vi "update_json_by_inserting_array.vi"(9 "json_to_insert_to_array(from recursive output)":string, 10 "ori_json_array":string[](array[string]), 11 "original_json":string) -> (3 "<JSON>输出":string)   [LabVIEW 2020]
uses:
  <vilib>/JDP Science/JSONtext/support/Format JSON Array Text.vi
  <vilib>/JDP Science/JSONtext/JSONtext.lvlib
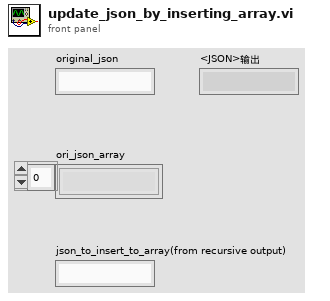
[diagram p1: front panel]
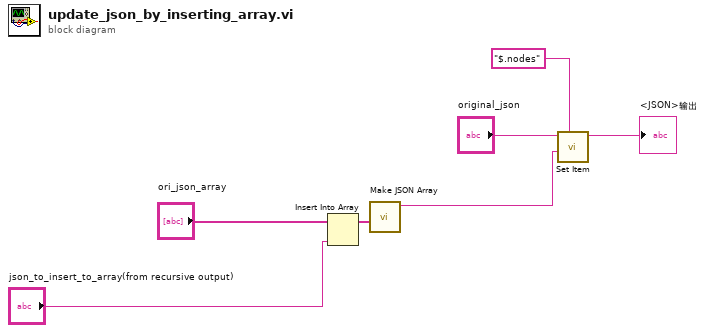
[diagram p0: block diagram]
diagram:
  n1 = Insert Into Array(array="ori_json_array", new element="json_to_insert_to_array(from recursive output)") -> (w2:string[])  [unwired: 1 in]
  n2 = call <vilib>:"Make JSON Array.vi"("JSON Elements"=w2) -> ("<JSON>"=w1:string)  [unwired: 9 in, 1 out]
  n3 = call <vilib>:"Set Item.vi"("$Path or Item Name"="$.nodes", "JSON to Insert"=w1, "JSON"="original_json") -> ("<JSON>"=→"<JSON>输出":string)  [unwired: 5 in, 2 out]
